vi "FT_Read_EEPROM_User_Area.vi"(0 "Handle":u32) -> (1 "FT_Status":u32(ring) items=["FT_OK", "FT_INVALID_HANDLE", "FT_DEVICE_NOT_FOUND", "FT_DEVICE_NOT_OPENED", "FT_IO_ERROR", "FT_INSUFFICIENT_RESOURCES", "FT_INVALID_PARAMETER", "FT_INVALID_BAUD_RATE", "FT_DEVICE_NOT_OPENED_FOR_ERASE", "FT_DEVICE_NOT_OPENED_FOR_WRITE", "FT_FAILED_TO_WRITE_DEVICE", "FT_EEPROM_READ_FAILED", "FT_EEPROM_WRITE_FAILED", "FT_EEPROM_ERASE_FAILED", "FT_EEPROM_NOT_PRESENT", "FT_EEPROM_NOT_PROGRAMMED", "FT_INVALID_ARGS", "FT_NOT_SUPPORTED", "FT_OTHER_ERROR"], 2 "User Area Data":u8[](array[numeric]), 3 "Bytes Read":u32)   [LabVIEW 2019, in "D2XX_Functions.lvlib"]
uses:
  <userlib>/LevyLab/Relay Box/D2XX_Functions/D2XX_Functions.lvlib
  <userlib>/LevyLab/Relay Box/D2XX_Functions/i386/ftd2xx.dll
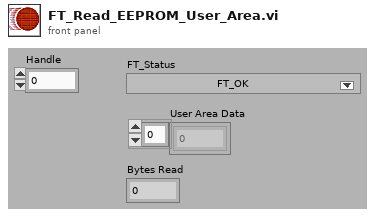
[diagram p1: front panel]
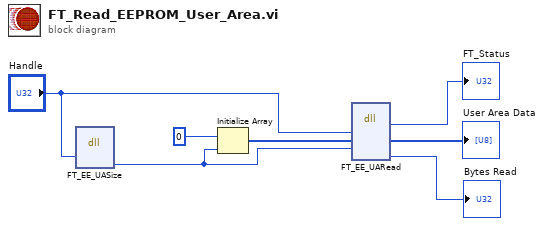
[diagram p0: block diagram]
diagram:
  n1 = dll-call lib="C:/Program Files (x86)/National Instruments/LabVIEW 2019/user.lib/LevyLab/Relay Box/D2XX_Functions/i386/FTD2XX.dll" fn="FT_EE_UASize"("Handle"="Handle") -> ("UASize"=w2:u32)  [unwired: 6 in, 2 out]
  n2 = Initialize Array(u16 0, w2) -> (w6:u16[])
  n3 = dll-call lib="C:/Program Files (x86)/National Instruments/LabVIEW 2019/user.lib/LevyLab/Relay Box/D2XX_Functions/i386/FTD2XX.dll" fn="FT_EE_UARead"("Handle"="Handle", "Buffer"=w6, "BytesToRead"=w2) -> ("FT_Status"=→"FT_Status":u32, "Buffer"=→"User Area Data":u8[], "BytesRead"=→"Bytes Read":u32)  [unwired: 6 in, 2 out]
